vi "Finish.vi"   [LabVIEW 2019]
doc: "This VI is called just before exiting. It is expected to close I/O refnum, save collected data, etc."
uses:
  <vilib>/Rock Robotics/WPI/Utilities/WPI_GetSetVariantRefNum.vi
types:
  T1 = typedef "WPI_JoystickDevRef.ctl" = cluster{"Device":T2}
  T2 = typedef "WPI_JoystickDeviceEnum.ctl" = enum16{"USB 0", "USB 1", "USB 2", "USB 3", "USB 4", "USB 5"}
  T3 = typedef "WPI_RobotDriveDevRef.ctl" = cluster{"DevStatus":errorcluster, "Motors[]":T4[], "Square Inputs":bool, "Max Output":dbl}
  T4 = typedef "WPI_MotorControlDeviceRef.ctl" = cluster{"DeviceStatus":errorcluster, "Type":T5, "PWM":cluster{"PWM Channel":T6, "DeadBand":T7}, "CAN":cluster{"Device Number":u8, "SetOutput VI Ref":variant, "GetOutput VI Ref":variant, "Enable VI Ref":variant, "Disable VI Ref":variant, "Data":variant}, "Invert":bool, "DIO PWM":cluster{"PWM \"Enable\" Channel":T6, "DIOChannel":T8, "PWM Rate":dbl}}
  T5 = typedef "WPI_MotorControlType.ctl" = enum16{"PWM", "CAN", "DIO PWM"}
  T6 = typedef "FPGA_DIOPWMChannel.ctl" = enum8{"PWM 0", "PWM 1", "PWM 2", "PWM 3", "PWM 4", "PWM 5", "PWM 6", "PWM 7", "PWM 8", "PWM 9", "PWM MXP 0", "PWM MXP 1", "PWM MXP 2", "PWM MXP 3", "PWM MXP 4", "PWM MXP 5", "PWM MXP 6", "PWM MXP 7", "PWM MXP 8", "PWM MXP 9", "Invalid"}
  T7 = typedef "WPI_PWMDeadband.ctl" = cluster{"Name":string, "maxPositivePwm":i32, "minPositivePwm":i32, "centerPwm":i32, "maxNegativePwm":i32, "minNegativePwm":i32, "angularRange":u16}
  T8 = typedef "FPGA_DIOChannel.ctl" = enum8{"DIO 0", "DIO 1", "DIO 2", "DIO 3", "DIO 4", "DIO 5", "DIO 6", "DIO 7", "DIO 8", "DIO 9", "DIO MXP 0", "DIO MXP 1", "DIO MXP 2", "DIO MXP 3", "DIO MXP 4", "DIO MXP 5", "DIO MXP 6", "DIO MXP 7", "DIO MXP 8", "DIO MXP 9", "DIO MXP 10", "DIO MXP 11", "DIO MXP 12", "DIO MXP 13", "DIO MXP 14", "DIO MXP 15", "SPI Port CS1", "SPI Port CS2", "SPI Port CS3", "SPI Port MISO", "SPI Port MOSI", "Invalid"}
  T9 = typedef "WPI_SolenoidDevRef.ctl" = cluster{"DevStatus":errorcluster, "Pneumatics Control Module":u8, "Forward Solenoid Channel":T10, "Reverse Solenoid Channel":T10}
  T10 = typedef "WPI_SolenoidChannel.ctl" = enum8{"Solenoid 0", "Solenoid 1", "Solenoid 2", "Solenoid 3", "Solenoid 4", "Solenoid 5", "Solenoid 6", "Solenoid 7", "Invalid"}
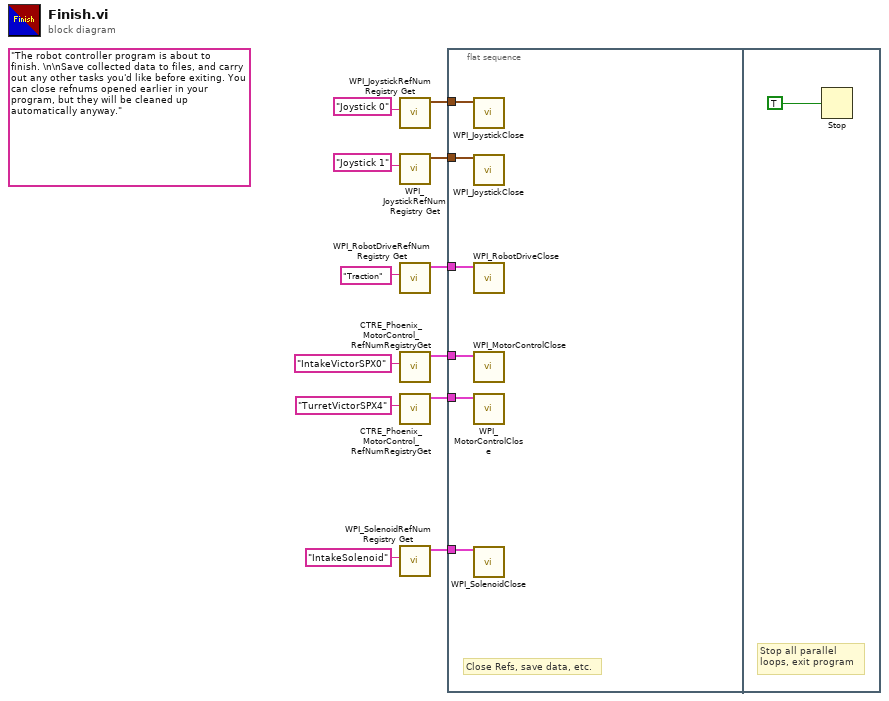
[diagram p0: block diagram]
diagram:
  (unwired) "The robot controller program is about to finish. \n\nSave collected data to files, and carry out any other tasks you'd like before exiting. You can close refnums opened earlier in your program, but they will be cleaned up automatically anyway."
  n1 = call <vilib>:"WPI_JoystickRefNum Registry Get.vi"("refnum name"="Joystick 0") -> ("JoystickDevRef"=w9:T1)  [unwired: 1 in, 9 out]
  n2 = call <vilib>:"WPI_JoystickRefNum Registry Get.vi"("refnum name"="Joystick 1") -> ("JoystickDevRef"=w3:T1)  [unwired: 1 in, 9 out]
  n3 = call <vilib>:"WPI_RobotDriveRefNum Registry Get.vi"("refnum name"="Traction") -> ("RobotDriveDevRef"=w10:T3)  [unwired: 1 in, 9 out]
  n4 = call <vilib>:"CTRE_Phoenix_MotorControl_RefNumRegistryGet.vi"("refnum name"="IntakeVictorSPX0") -> ("PhoenixMotorControlDevRef"=w8:T4)  [unwired: 9 in, 1 out]
  n5 = call <vilib>:"CTRE_Phoenix_MotorControl_RefNumRegistryGet.vi"("refnum name"="TurretVictorSPX4") -> ("PhoenixMotorControlDevRef"=w1:T4)  [unwired: 9 in, 1 out]
  n6 = call <vilib>:"WPI_SolenoidRefNum Registry Get.vi"("refnum name"="IntakeSolenoid") -> ("SolenoidDevRef"=w7:T9)  [unwired: 9 in, 1 out]
  n7 = flat-sequence {
    tunnel: w10 -> [w18]
    tunnel: w9 -> [w17]
    tunnel: w8 -> [w16]
    tunnel: w7 -> [w15]
    tunnel: w3 -> [w14]
    tunnel: w1 -> [w13]
    frame #0 {
      # "Close Refs, save data, etc."
      n8 = call <vilib>:"WPI_JoystickClose.vi"("JoystickDevRef"=w17) -> ()  [unwired: 11 out]
      n9 = call <vilib>:"WPI_JoystickClose.vi"("JoystickDevRef"=w14) -> ()  [unwired: 11 out]
      n10 = call <vilib>:"WPI_RobotDriveClose.vi"("RobotDriveDevRef"=w18) -> ()  [unwired: 1 in, 10 out]
      n11 = call <vilib>:"WPI_MotorControlClose.vi"("MotorControlDevRef"=w16) -> ()  [unwired: 10 in, 1 out]
      n12 = call <vilib>:"WPI_MotorControlClose.vi"("MotorControlDevRef"=w13) -> ()  [unwired: 10 in, 1 out]
      n13 = call <vilib>:"WPI_SolenoidClose.vi"("SolenoidDevRef"=w15) -> ()  [unwired: 10 in, 1 out]
    }
    frame #1 {
      # "Stop all parallel\nloops, exit program"
      n14 = Stop(stop? (T)=TRUE ("Quit")) -> ()
    }
  }
